vi "Test Counter.vi"() -> ()   [LabVIEW 2016, in "BNT_DAQmx.lvlib"]
uses:
  BNT_DAQmx.lvlib
panel:
  out "Frequency SV":dbl[unit]
  out "Frequency Calc":dbl[unit]
  in  "Frequeny":dbl[unit]=10.0
  in  "Stop":bool
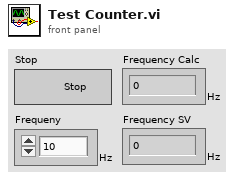
[diagram p1: front panel]
types:
  T1 = cluster{"Read Access":enum8{"Allowed", "Required", "None"}, "Write Access":enum8{"Allowed", "Required", "None"}}
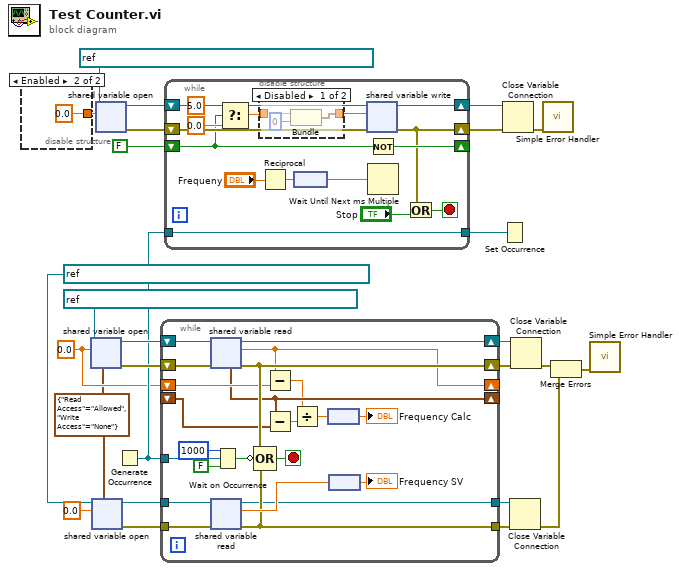
[diagram p0: block diagram]
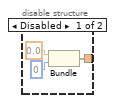
[diagram p2: hidden frame]
diagram:
  w11 = 0.0
  w8 = T1 {"Read Access"=enum."Allowed", "Write Access"=enum."None"} ("access")
  n1 = disable-structure shown="Enabled" {
    disable-tunnel: [w27 0.0] -> w10
    frame Disabled {
      n2 = Bundle(0.0, 0) -> (w27:cluster{dbl, i32})  [unwired: 1 in]
    }
    frame Enabled {
    }
  }
  n3 = shared-variable-open(refnum<k21> "ni.var.psp://localhost/EQCR-SV/myDAQ_Counter0" ("shared variable refnum in"), w11, w8) -> (w18:refnum<k21>, w17:errorcluster)  [unwired: 1 in]
  n4 = shared-variable-open(refnum<k21> "ni.var.psp://localhost/EQCR-SV/myDAQ_Frequency0" ("shared variable refnum in"), 0.0, w8) -> (w6:refnum<k21>, w5:errorcluster)  [unwired: 1 in]
  n5 = shared-variable-open(refnum<k21> "ni.var.psp://localhost/EQCR-SV/myDAQ_Set-AO_0" ("shared variable refnum in"), w10) -> (w25:refnum<k21>, w22:errorcluster)  [unwired: 2 in]
  n6 = Generate Occurrence() -> (w16:refnum<k4>)
  n7 = while {
    shift-right: [w51] -> w13
    shift-left: w18 -> [w53]
    shift-right: [w46] -> w12
    shift-left: w17 -> [w52]
    tunnel: w16 -> [w50]
    shift-right: [w43] -> _
    shift-left: w11 -> [w44]
    shift-right: [w42] -> _
    shift-left: _ -> [w41]
    tunnel: w6 -> [w36]
    tunnel: w5 -> [w35]
    tunnel: [w33] -> w4
    tunnel: [w32] -> w3
    stop <- w45 stop-if-true
    n8 = shared-variable-read(w53, w52) -> (w51:refnum<k21>, w46:errorcluster, w43:dbl, w42:timestamp)
    n9 = shared-variable-read(w36, w35) -> (w32:refnum<k21>, w33:errorcluster, w34:dbl)  [unwired: 1 out]
    n10 = Wait on Occurrence(1:FALSE ("ignore previous (T)"), 2:w50, 3:1000 ("ms timeout (-1)")) -> (0:w47:bool)
    n11 = Compound Arithmetic op=OR(w46, invert w47, w33) -> (w45:bool)
    n12 = Subtract(x=w43, y=w44) -> (x-y=w40:dbl)
    n13 = Subtract(x=w42, y=w41) -> (x-y=w39:dbl)
    n14 = Divide(x=w40, y=w39) -> (x/y=w38:dbl)
    n15 = node(w38) -> (→"Frequency Calc":dbl[unit])
    n16 = node(w34) -> (→"Frequency SV":dbl[unit])
  }
  n17 = while {
    shift-right: [w68] -> w24
    shift-left: w25 -> [w69]
    shift-right: [w57] -> w23
    shift-left: w22 -> [w67]
    shift-right: [w65] -> _
    shift-left: FALSE -> [w62]
    tunnel: w16 -> [w56]
    tunnel: [w56] -> w15
    stop <- w58 stop-if-true
    n18 = Select(t=5.0, s=w62, f=0.0) -> (s? t:f=w54:dbl)
    n19 = disable-structure shown="Disabled" {
      disable-tunnel: [w72 w73] -> w55
      disable-tunnel: w54 -> [w71 w73]
      frame Disabled {
        n20 = Bundle("f"=w71, 0) -> (w72:cluster{"f":dbl, i32})  [unwired: 1 in]
      }
      frame Enabled {
      }
    }
    n21 = Reciprocal(x="Frequeny") -> (1/x=w59:dbl[unit])
    n22 = node(w59) -> (w60:dbl)
    n23 = shared-variable-write(w69, w67, w55) -> (w68:refnum<k21>, w57:errorcluster)
    n24 = Not(x=w62) -> (.not. x?=w65:bool)
    n25 = Wait Until Next ms Multiple(millisecond multiple=w60) -> ()  [unwired: 1 out]
    n26 = Or(x=w57, y="Stop") -> (x .or. y?=w58:bool)
  }
  n27 = Set Occurrence(w15) -> ()
  n28 = Close Variable Connection(8:w23, 11:w24) -> (0:w20:errorcluster)
  n29 = Close Variable Connection(8:w4, 11:w3) -> (0:w1:errorcluster)
  n30 = Close Variable Connection(8:w12, 11:w13) -> (0:w14:errorcluster)
  n31 = call <vilib>:"Simple Error Handler.vi"("error in (no error)"=w20) -> ()  [unwired: 4 in, 5 out]
  n32 = Merge Errors(w14, w1) -> (w2:errorcluster)
  n33 = call <vilib>:"Simple Error Handler.vi"("error in (no error)"=w2) -> ()  [unwired: 4 in, 5 out]
